vi "RT-Remote-v4.vi"() -> ()   [LabVIEW 2017]
uses:
  <vilib>/rvi/interface/nirviOpenFPGA/nirviOpenFPGA.xnode
  <vilib>/rvi/interface/nirviMethod/nirviMethod.xnode
  <vilib>/rvi/interface/nirviCloseFPGA/nirviCloseFPGA.xnode
  <vilib>/rvi/interface/nirviReadWriteControl/nirviReadWriteControl.xnode
  <vilib>/rvi/interface/Simulation/niFpgaSimulationCallBeginRW.vi
  <vilib>/rvi/errors/niLvFpgaAdjustHostInterfaceError.vi
  <vilib>/FPGAPlugInAG/Dynamic/niLvFpga_WriteFifo_Dynamic.vi
  <vilib>/rvi/errors/niLvFpgaMergeErrorWithErrorCode.vi
  <vilib>/FPGAPlugInAG/Dynamic/niLvFpga_Reset_Dynamic.vi
  <vilib>/nisyscfg/nisyscfg.lvlib
  NiFpgaLv.dll
  State Machine.vi
  <vilib>/FPGAPlugInAG/cRIO-9068/niLvFpga_Open_cRIO-9068.vi
  <vilib>/rvi/interface/common/dynamic/niFpgaDynamicAddResources.vi
  <vilib>/FPGAPlugInAG/Dynamic/niLvFpga_Close_Dynamic.vi
  <vilib>/rvi/interface/nirviMethod/StockFPGA_InlinedMethodWaitForSingleIRQ.vi
  <vilib>/FPGAPlugInAG/Dynamic/niLvFpga_WaitOnIrq_Dynamic.vi
  <vilib>/FPGAPlugInAG/Dynamic/niLvFpga_AcknowledgeIrq_Dynamic.vi
  <vilib>/FPGAPlugInAG/Dynamic/niLvFpga_ReadFifo_Dynamic.vi
  FPGA Bitfiles/NIcRIOFPGA_OMX-TFPGA_FPGAoptimizeperf_aoKWFa4HCLY.lvbitx
panel:
  out "error before tcp read":errorcluster
  out "Error after tcp read":errorcluster
  in  "Reset RT":bool
  out "cluster 406":T1
  out "output cluster 406":cluster{u16, u16}
  out "data out 200":string
  out "data out 100":string
  out "RT-host IP":string="10.6.19.12"
  out "Master Computer IP":string="10.6.19.11"
  out "UDP refresh rate":u16=100
  out "UDP receiving port":i32=6666
  out "UDP sending port":u16=6666
  out "Run Status reporter":bool=TRUE
  out "JSON Command":string
  out "Command \nConnection Port":u16=5000
  out "error out":errorcluster
  out "RT-host Action State":T2(ring)
  out "RT-host\nMain State":T3(ring)
  out "JSON string":string
  in  "Temperature Units (C) 2":u16(ring) items=["Celsius", "Fahrenheit", "Kelvin", "Rankine"]
  in  "ThermocoupleType 2":u16(ring)=2 items=["B", "E", "J", "K", "R", "S", "T", "N", "IC (C)", "IC (F)", "Therm."]
  out "Data sender Error out":errorcluster caption="error out"
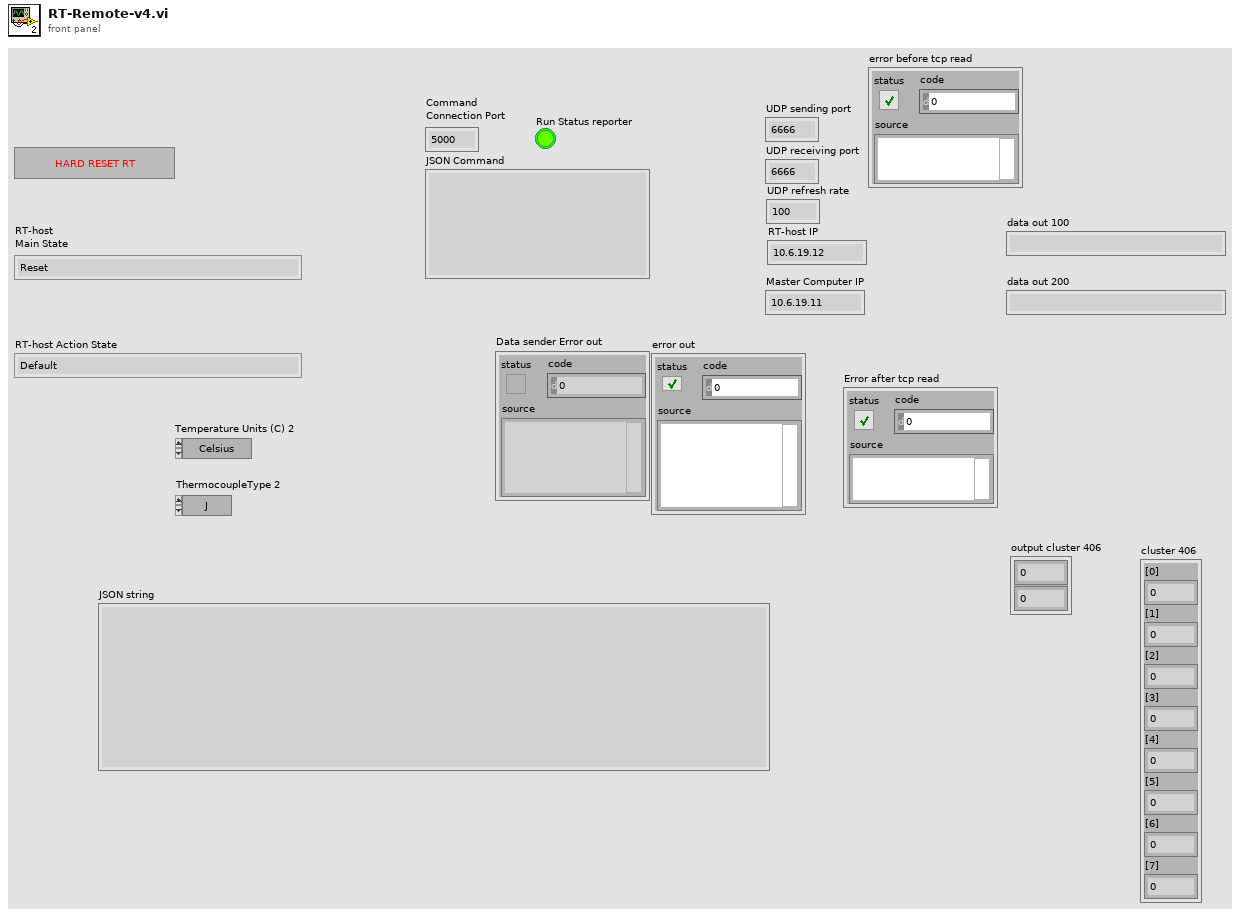
[diagram p1: front panel]
types:
  T1 = cluster{"[0]":u16, "[1]":u16, "[2]":u16, "[3]":u16, "[4]":u16, "[5]":u16, "[6]":u16, "[7]":u16}
  T2 = enum16{"Default", "Sending Digitals", "Sending Analogue", "Writing Digitals", "Writing Analogue", "Updating Repetitions", "Updating Indexes", "Init Profile", "Triggering Experiment", "Take Snap", "Flushing FIFOs", ""}
  T3 = enum16{"Reset", "Start", "Configuring", "Waiting Connection", "Idle", "Verifying FPGA state", "Sending Sync Command", "Sending Async Command", "Aborted", "Shutdown"}
  T4 = cluster{"Command":u16, "Message Length":u16, "Number of Messages":u32}
  T5 = enum16{"Reset", "Start", "Configuring", "Waiting Connection", "Idle", "Verifying FPGA state", "Sending Sync Command", "Sending Async Command", "Aborted", "Shutdown", "Send Error", ""}
  T6 = cluster{"FPGA Main State":u8, "FPGA Action State":u8, "Digitals":u16, "Analogue 0":i16, "Analogue 1":i16, "Analogue 2":i16, "Analogue 3":i16, "Temperature 0":sgl, "Temperature 1":sgl, "Temperature 2":sgl, "Temperature 3":sgl, "Error Description":string, "Error Status":bool, "Error code":i32, "RT-host Main State":u8, "RT-host Action State":u8, "Aborted":bool, "Interlock":bool, "Event":string}
  T7 = enum8{"Default", "Start", "Configuring", "Idle", "Aborted", "Running Action", "ShutDown"}
  T8 = enum8{"Default", "Executing Experiment", "Transfering Digitals", "Transfering Analogues", "Writing Indexes", "Writing Digitals", "Writing Analogue", "Taking Snap", "Flushing FIFOs", "Updating Repetitions"}
  T9 = cluster{"Mod6/CJC":fxp<+/-,24,-2>, "Mod6/TC0":fxp<+/-,24,-2>, "Mod6/TC1":fxp<+/-,24,-2>, "Mod6/TC2":fxp<+/-,24,-2>, "Mod6/TC3":fxp<+/-,24,-2>, "Mod6/Autozero":fxp<+/-,24,-2>}
  T10 = cluster{"Command":u8, "Message Length":u16, "Number of Messages":u32}
  T11 = enum16{"Standard", "Buffered", "CRLF", "Immediate"}
  T12 = cluster{"Command":u8, "Message Length":u16, "Number of Messages":u16}
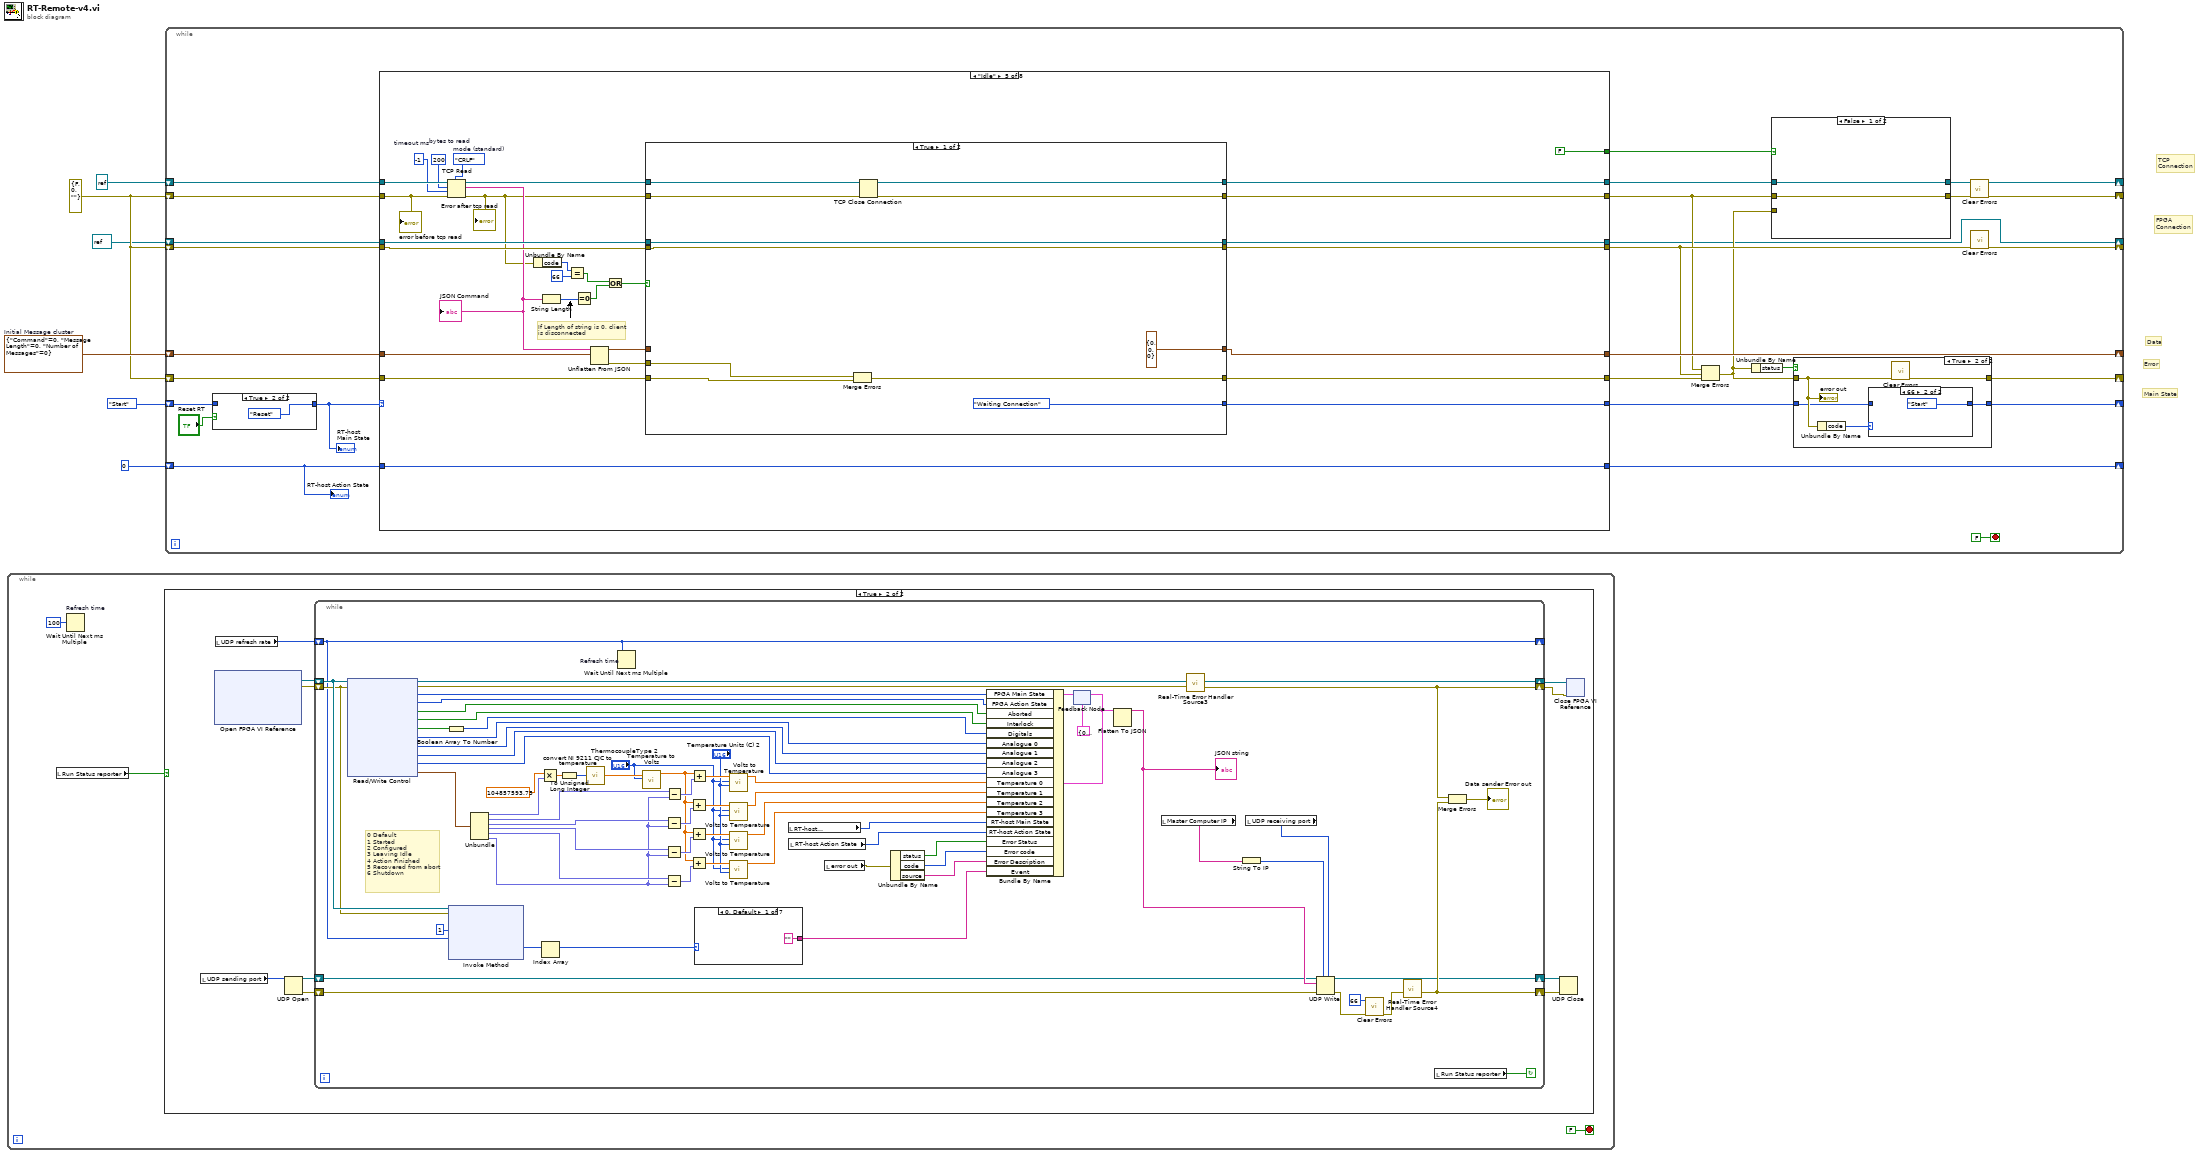
[diagram p0: block diagram]
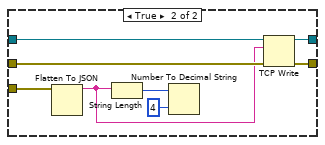
[diagram p3: hidden frame]
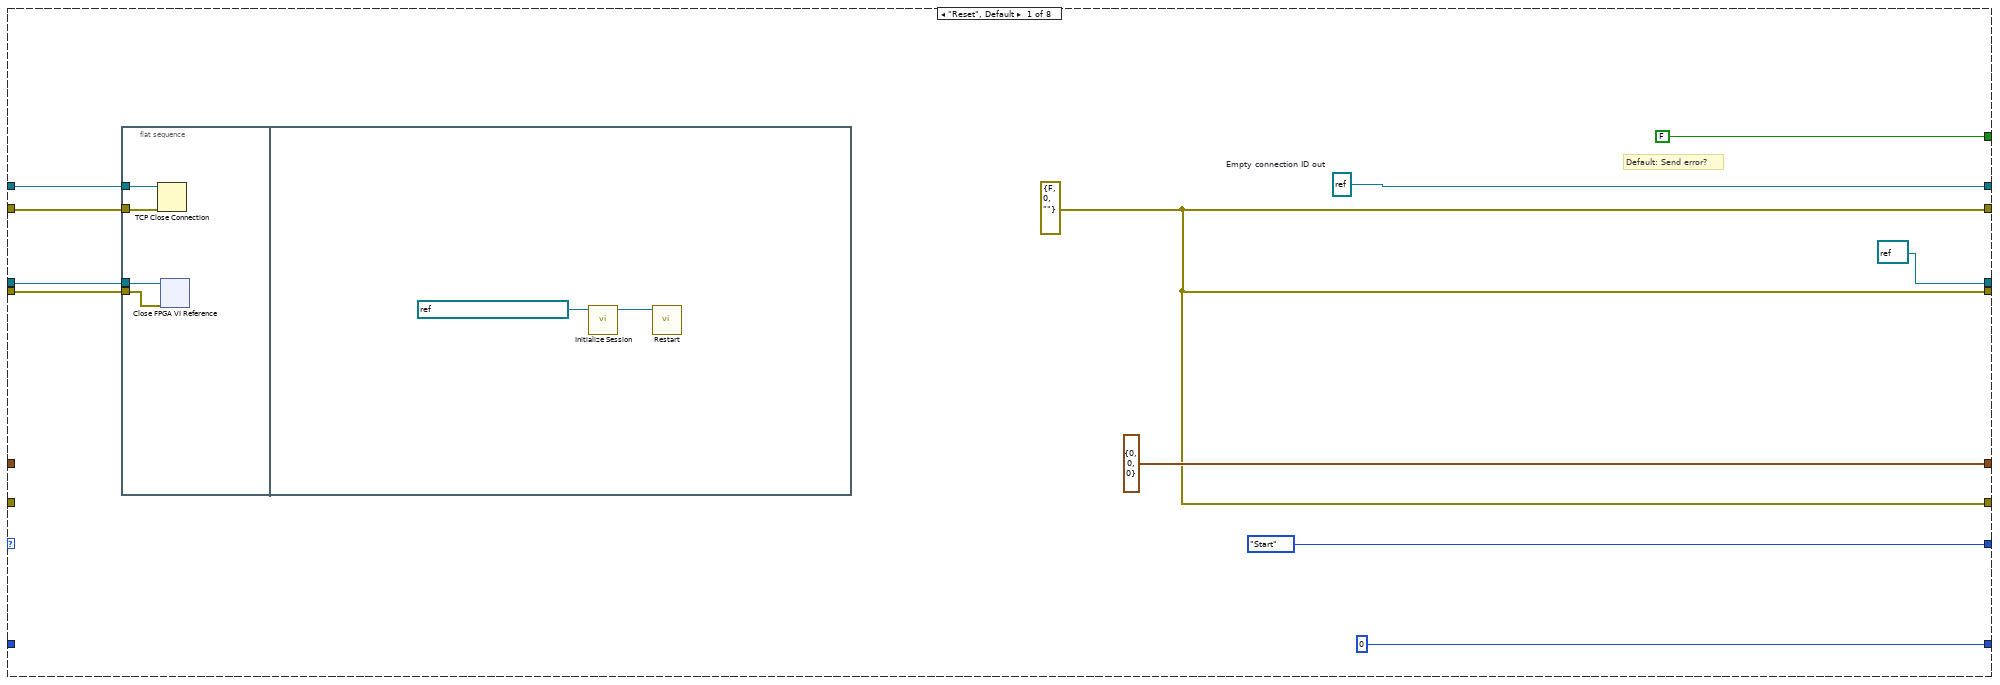
[diagram p6: hidden frame]
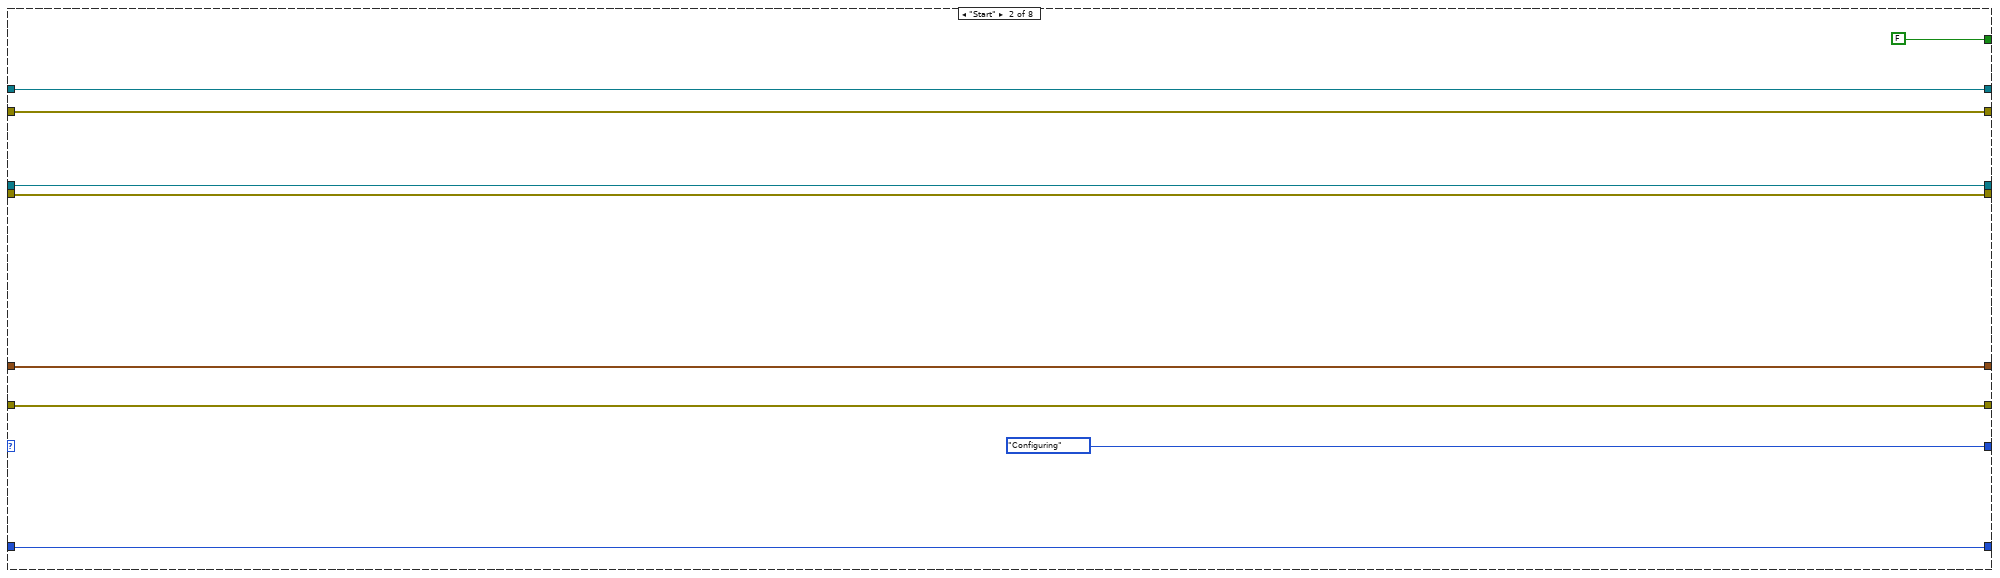
[diagram p7: hidden frame]
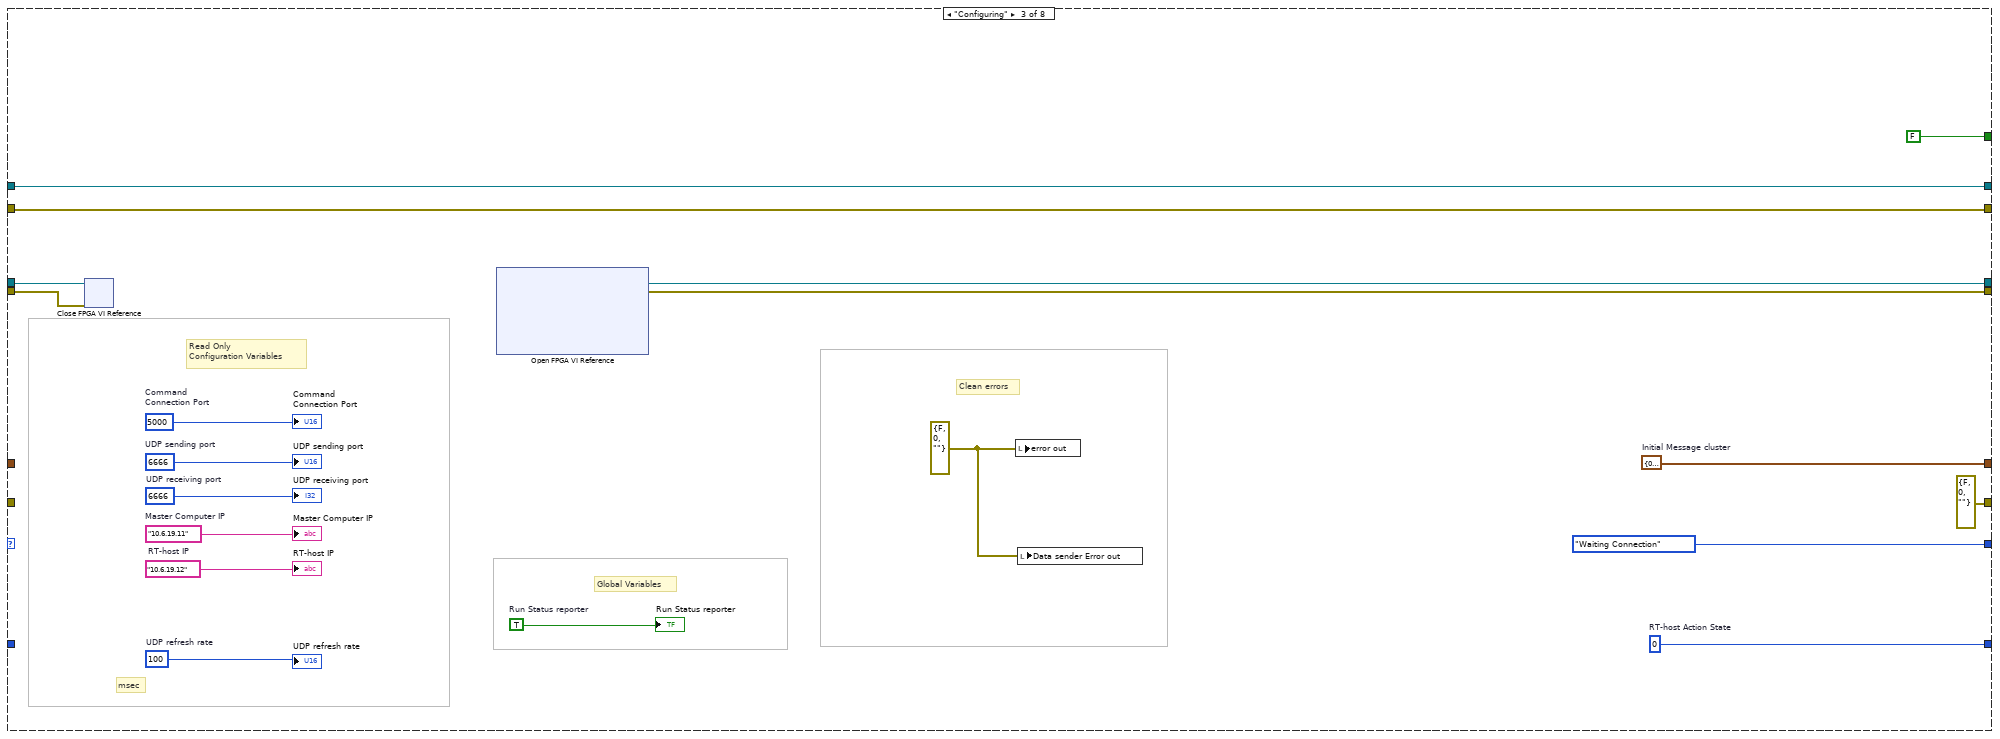
[diagram p8: hidden frame]
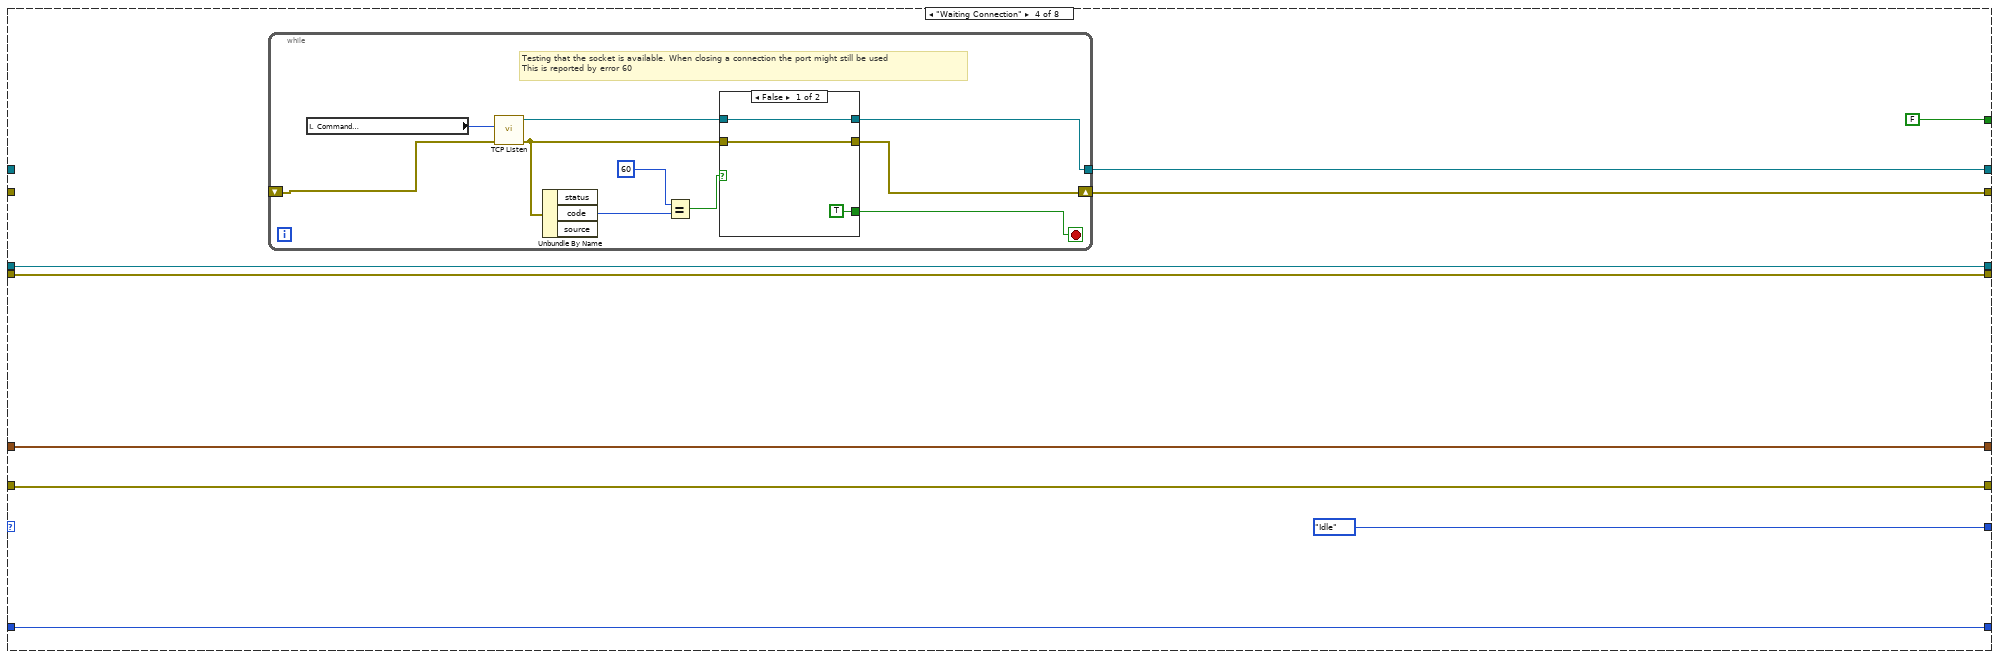
[diagram p9: hidden frame]
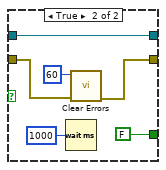
[diagram p10: hidden frame]
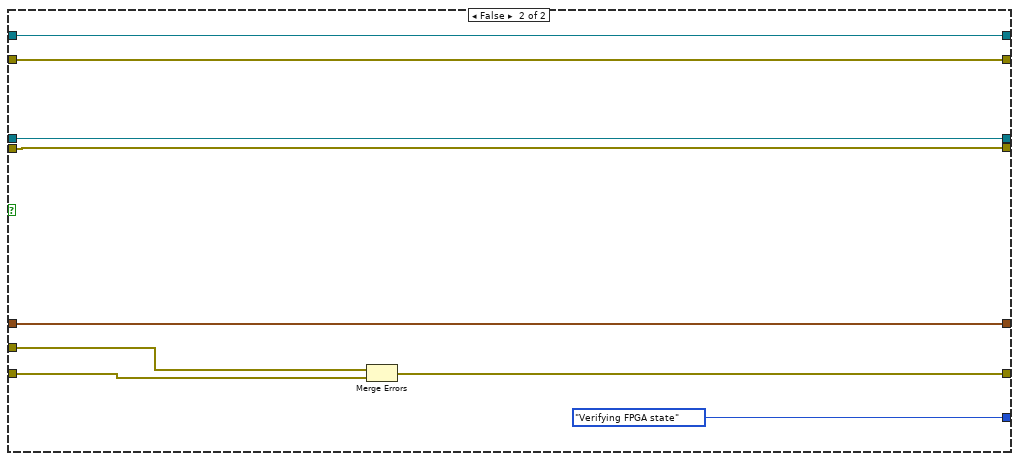
[diagram p11: hidden frame]
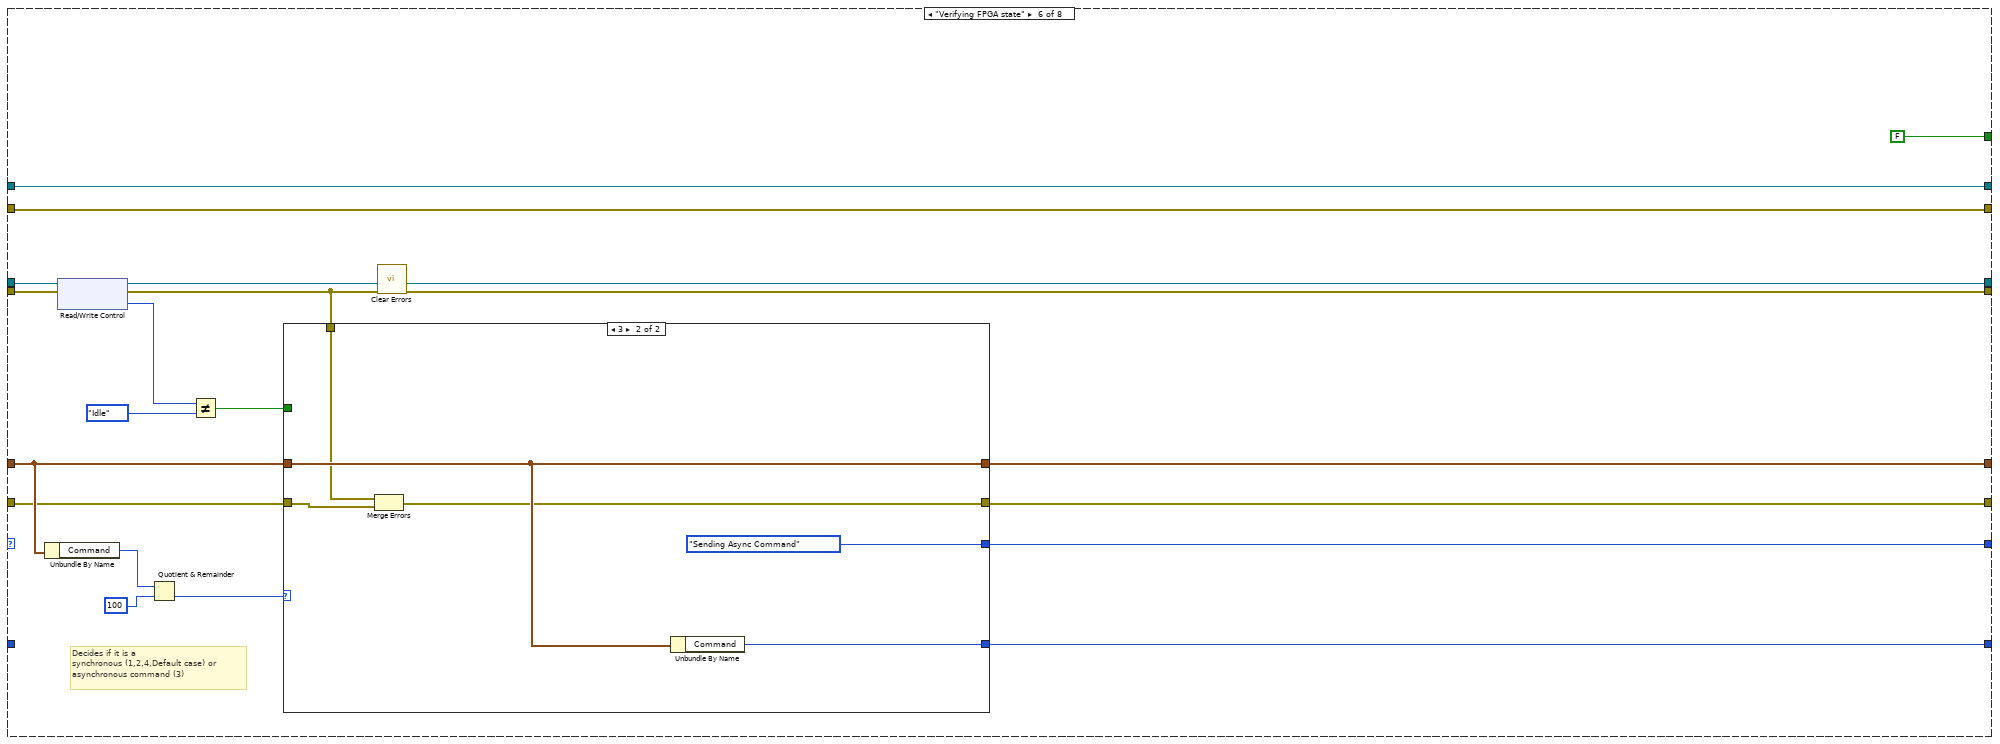
[diagram p12: hidden frame]
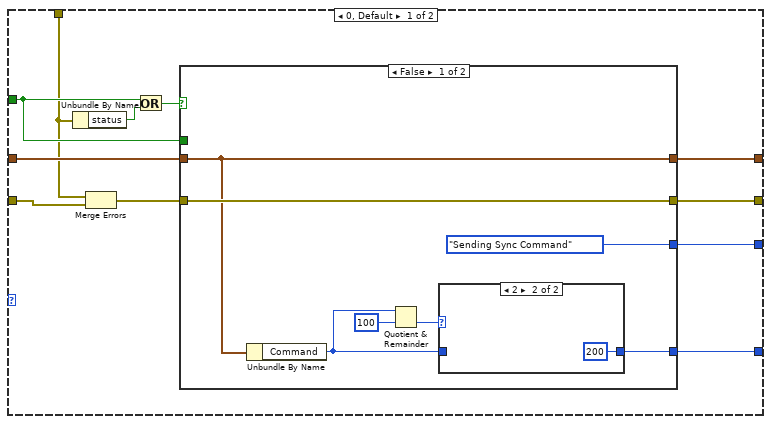
[diagram p13: hidden frame]
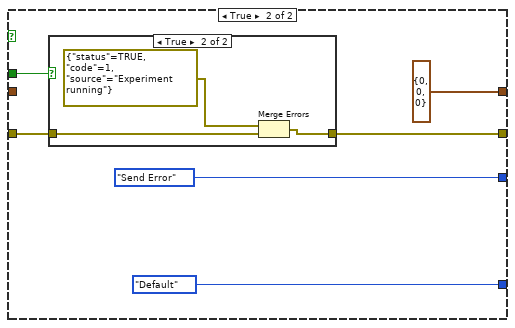
[diagram p15: hidden frame]
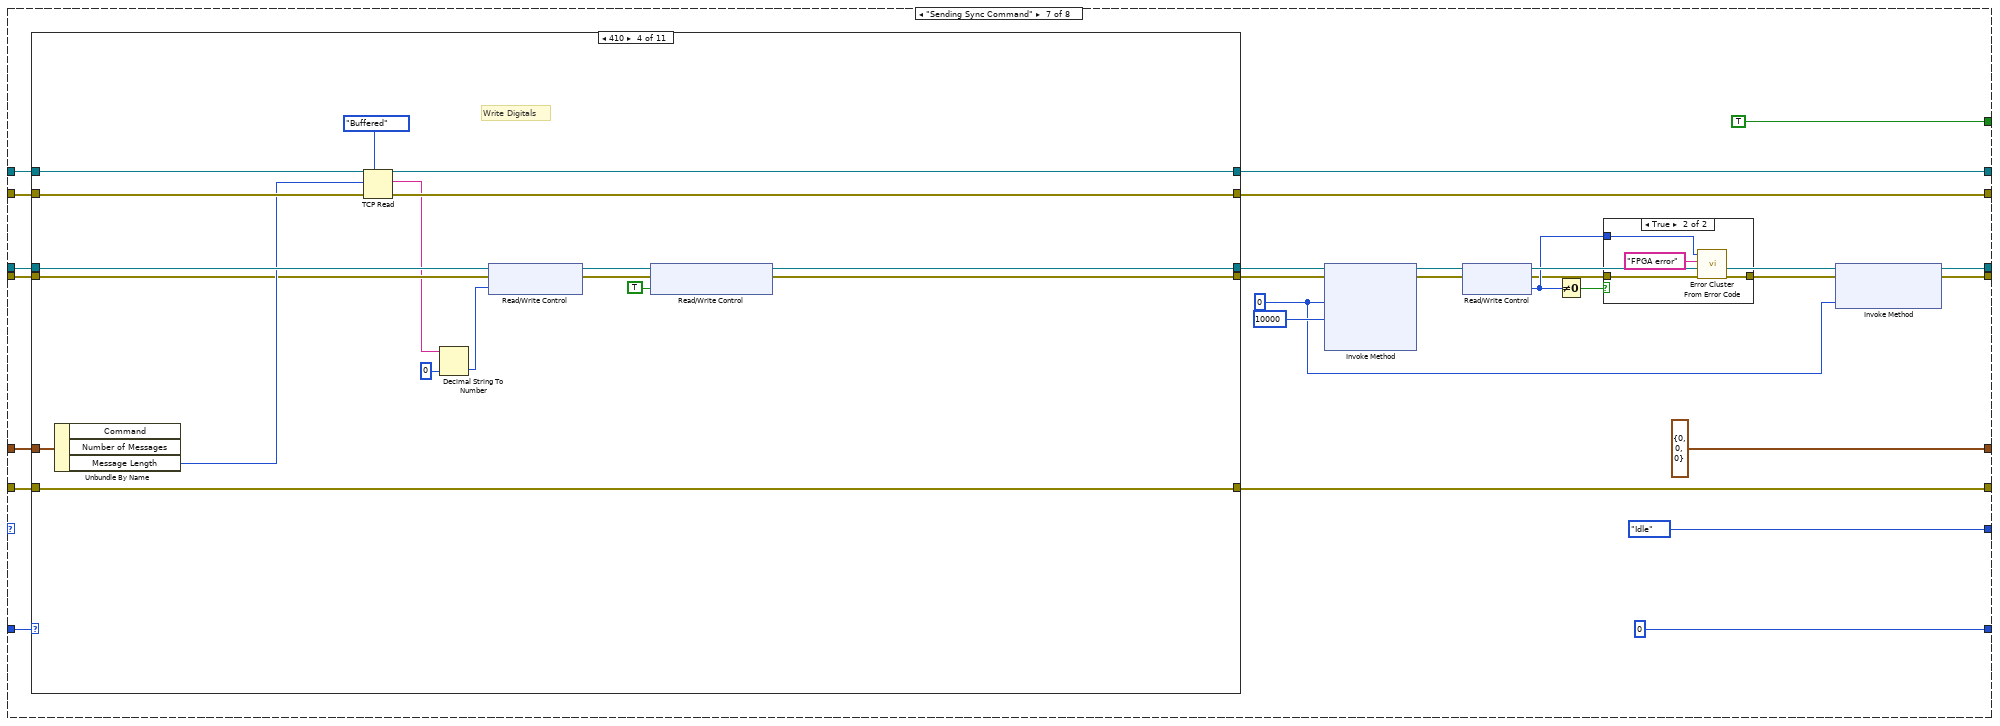
[diagram p17: hidden frame]
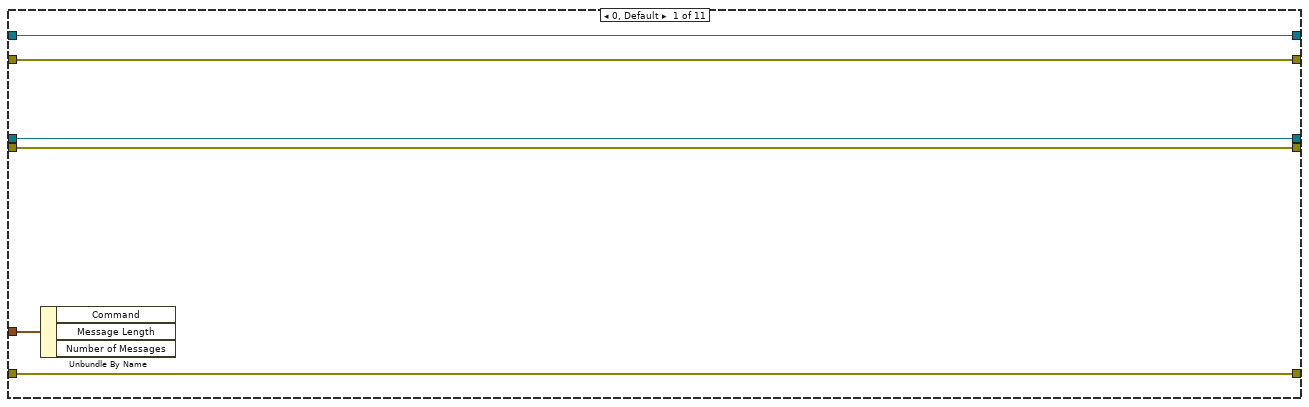
[diagram p19: hidden frame]
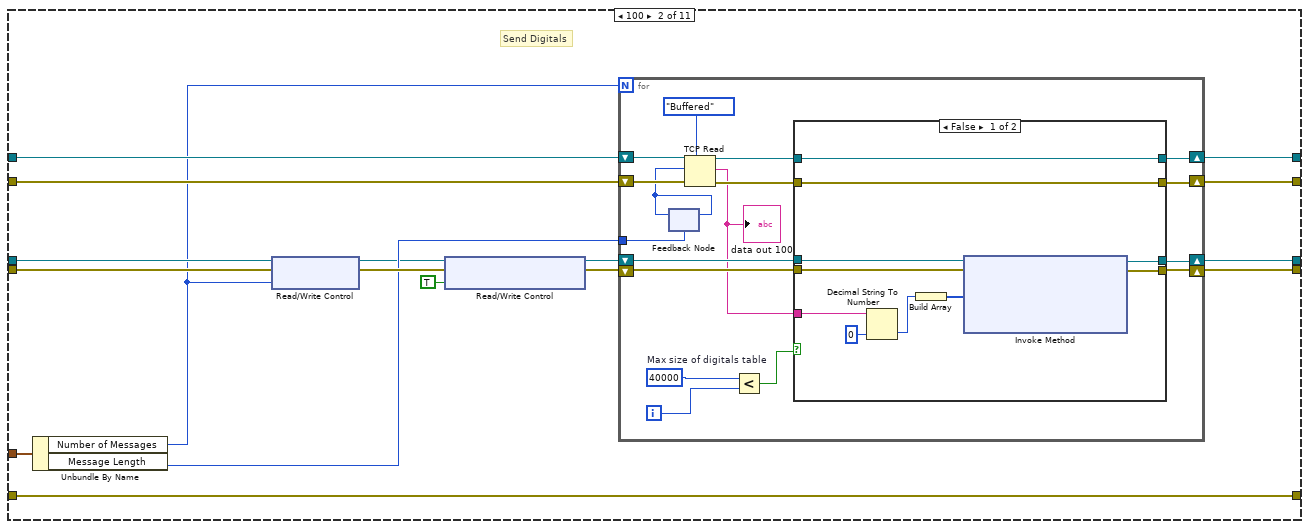
[diagram p20: hidden frame]
diagram:
  w2 = errorcluster {"status"=FALSE, "code"=0, "source"=""} ("error out")
  w5 = T4 {"Command"=0, "Message Length"=0, "Number of Messages"=0}  # Initial Message cluster
  # "Main State"
  # "Error"
  # "Data"
  # "FPGA\nConnection"
  # "TCP\nConnection"
  n1 = while {
    stop <- FALSE stop-if-true
    n2 = local read "Run Status reporter"() -> (w7:bool)
    n3 = Wait Until Next ms Multiple "Refresh time"(millisecond multiple=u32 100) -> ()  [unwired: 1 out]
    n4 = case shown="True" w7 {
      frame False {
      }
      frame True {
        n5 = local read "UDP sending port"() -> (w11:u16)
        n6 = xnode "Open FPGA VI Reference"() -> ("FPGA VI Reference Out"=w12:refnum<k20>, "error out"=w13:errorcluster)  [unwired: 2 in]
        n7 = local read "UDP refresh rate"() -> (w10:u16)
        n8 = UDP Open(11:w11) -> (port=w17:refnum<k16>, 0:w14:errorcluster)  [unwired: 4 in, 1 out]
        n9 = while {
          shift-right: [w84] -> w16
          shift-left: w17 -> [w22]
          shift-right: [w85] -> w18
          shift-left: w14 -> [w21]
          shift-right: [w56] -> w19
          shift-left: w12 -> [w30]
          shift-right: [w83] -> w15
          shift-left: w13 -> [w26]
          shift-right: [w24] -> _
          shift-left: w10 -> [w24]
          stop <- w32 continue-if-true
          # "0 Default\n1 Started\n2 Configured\n3 Leaving Idle \n4 Action Finished\n5 Recovered from abort\n6 Shutdown"
          n10 = xnode "Read/Write Control"("FPGA VI Reference In"=w30, "error in"=w26) -> ("FPGA VI Reference Out"=w56:refnum<k20>, "error out"=w55:errorcluster, "Main State"=w44:T7, "Action State"=w45:T8, "Aborted"=w34:bool, "Interlock"=w57:bool, "Digitals"=w80:bool[], "Analogue 0"=w47:i16, "Analogue 1"=w48:i16, "Analogue 2"=w49:i16, "Analogue 3"=w50:i16, "Temperatures array"=w58:T9)
          n11 = Boolean Array To Number(Boolean array=w80) -> (number=w46:u16)
          n12 = xnode "Invoke Method"("FPGA VI Reference In"=w30, "error in"=w26, "Number of Elements"=u32 1, "Timeout (ms)"=w24) -> ("Data"=w28:u8[])  [unwired: 3 out]
          n13 = Unbundle(w58) -> ("Mod6/CJC"=w76:fxp<+/-,24,-2>, "Mod6/TC0"=w73:fxp<+/-,24,-2>, "Mod6/TC1"=w66:fxp<+/-,24,-2>, "Mod6/TC2"=w65:fxp<+/-,24,-2>, "Mod6/TC3"=w64:fxp<+/-,24,-2>, "Mod6/Autozero"=w63:fxp<+/-,24,-2>)
          n14 = Multiply(x=104857593.75 ("y"), y=w76) -> (x*y=w77:dbl)
          n15 = Index Array(array=w28) -> (element=w27:u8)  [unwired: 1 in]
          n16 = To Unsigned Long Integer(number=w77) -> (unsigned 32bit integer=w78:u32)
          n17 = call "convert NI 9211 CJC to temperature.vi"("CJC Channel"=w78) -> ("CJC Temperature (C)"=w79:sgl)
          n18 = Wait Until Next ms Multiple "Refresh time"(millisecond multiple=w24) -> ()  [unwired: 1 out]
          n19 = call "Temperature to Volts.vi"("ThermocoupleType"="ThermocoupleType 2", "Temperature"=w79) -> ("Thermocouple Voltage"=w59:sgl)  [unwired: 1 in, 4 out]
          n20 = Subtract(x=w66, y=w63) -> (x-y=w62:fxp<+/-,25,-1>)
          n21 = Subtract(x=w65, y=w63) -> (x-y=w61:fxp<+/-,25,-1>)
          n22 = Subtract(x=w64, y=w63) -> (x-y=w60:fxp<+/-,25,-1>)
          n23 = Subtract(x=w73, y=w63) -> (x-y=w72:fxp<+/-,25,-1>)
          n24 = Add(x=w59, y=w62) -> (x+y=w71:sgl)
          n25 = Add(x=w59, y=w61) -> (x+y=w70:sgl)
          n26 = Add(x=w59, y=w60) -> (x+y=w69:sgl)
          n27 = Add(x=w59, y=w72) -> (x+y=w74:sgl)
          n28 = case shown="0, Default" w27 {
            tunnel: ["" "started" "configured" "leaving idle" "done" "recovered from abort" "shutdown"] -> w25
            frame 0, Default {
            }
            frame 1 {
            }
            frame 2 {
            }
            frame 3 {
            }
            frame 4 {
            }
            frame 5 {
            }
            frame 6 {
            }
          }
          n29 = call <vilib>:"Volts to Temperature.vi"("Temperature Units"="Temperature Units (C) 2", "ThermocoupleType"="ThermocoupleType 2", "Thermocouple Voltage"=w71) -> ("Temperature"=w52:sgl)  [unwired: 4 out]
          n30 = call <vilib>:"Volts to Temperature.vi"("Temperature Units"="Temperature Units (C) 2", "ThermocoupleType"="ThermocoupleType 2", "Thermocouple Voltage"=w70) -> ("Temperature"=w53:sgl)  [unwired: 4 out]
          n31 = call <vilib>:"Volts to Temperature.vi"("Temperature Units"="Temperature Units (C) 2", "ThermocoupleType"="ThermocoupleType 2", "Thermocouple Voltage"=w69) -> ("Temperature"=w54:sgl)  [unwired: 4 out]
          n32 = call <vilib>:"Volts to Temperature.vi"("Temperature Units"="Temperature Units (C) 2", "ThermocoupleType"="ThermocoupleType 2", "Thermocouple Voltage"=w74) -> ("Temperature"=w51:sgl)  [unwired: 4 out]
          n33 = local read "RT-host\nMain State"() -> (w40:T3)
          n34 = local read "RT-host Action State"() -> (w39:T2)
          n35 = local read "error out"() -> (w38:errorcluster)
          n36 = Unbundle By Name(w38) -> ("status"=w37:bool, "code"=w36:i32, "source"=w35:string)
          n37 = feedback #1(T6 {"FPGA Main State"=0, "FPGA Action State"=0, "Digitals"=0, "Analogue 0"=0, "Analogue 1"=0, "Analogue 2"=0, "Analogue 3"=0, "Temperature 0"=0.0, "Temperature 1"=0.0, "Temperature 2"=0.0, "Temperature 3"=0.0, "Error Description"="", "Error Status"=FALSE, "Error code"=0, "RT-host Main State"=0, "RT-host Action State"=0, "Aborted"=FALSE, "Interlock"=FALSE, "Event"=""}) -> (w42:T6)
          n38 = Bundle By Name(cluster=w42, "FPGA Main State"=w44, "FPGA Action State"=w45, "Aborted"=w34, "Interlock"=w57, "Digitals"=w46, "Analogue 0"=w47, "Analogue 1"=w48, "Analogue 2"=w49, "Analogue 3"=w50, "Temperature 0"=w51, "Temperature 1"=w52, "Temperature 2"=w53, "Temperature 3"=w54, "RT-host Main State"=w40, "RT-host Action State"=w39, "Error Status"=w37, "Error code"=w36, "Error Description"=w35, "Event"=w25) -> (w41:T6)
          n39 = feedback-in #1(w41) -> ()
          n40 = Flatten To JSON(anything=w41) -> (JSON string=w31:string)  [unwired: 2 in, 1 out]
          "JSON string" <- w31
          n41 = local read "Master Computer IP"() -> (w33:string)
          n42 = call "Real-Time Error Handler Source3"("Error to Check"=w55) -> ("error out"=w83:errorcluster)  [unwired: 11 in, 3 out]
          n43 = String To IP(1:w33) -> (0:w23:u32)
          n44 = local read "UDP receiving port"() -> (w20:i32)
          n45 = UDP Write(address=w23, port or service name=w20, connection ID=w22, data in=w31, 8:w21) -> (error out=w87:errorcluster, 3:w84:refnum<k16>)  [unwired: 1 in]
          n46 = call <vilib>:"Clear Errors.vi"("error in (no error)"=w87, "specific error code to clear (0: all)"=66) -> ("error out"=w82:errorcluster)  [unwired: 4 in, 1 out]
          n47 = call "Real-Time Error Handler Source4"("Error to Check"=w82) -> ("error out"=w85:errorcluster)  [unwired: 11 in, 3 out]
          n48 = local read "Run Status reporter"() -> (w32:bool)
          n49 = Merge Errors(w83, w85) -> (→"Data sender Error out":errorcluster)
        }
        n50 = UDP Close(connection ID=w16, 8:w18) -> ()  [unwired: 2 out]
        n51 = xnode "Close FPGA VI Reference"("FPGA VI Reference In"=w19, "error in"=w15) -> ()  [unwired: 1 out]
      }
    }
  }
  n52 = while {
    shift-right: [w100] -> _
    shift-left: T5."Start" ("RT-host Main State") -> [w97]
    shift-right: [w105] -> _
    shift-left: refnum<k5> refnum ("connection ID out") -> [w122]
    shift-right: [w121] -> _
    shift-left: w5 -> [w120]
    shift-right: [w118] -> _
    shift-left: u16 0 ("RT-host Action State") -> [w115]
    shift-right: [w111] -> _
    shift-left: w2 -> [w117]
    shift-right: [w110] -> _
    shift-left: w2 -> [w116]
    shift-right: [w113] -> _
    shift-left: w2 -> [w114]
    shift-right: [w98] -> _
    shift-left: refnum<k20> refnum ("FPGA VI Reference Out") -> [w99]
    stop <- FALSE stop-if-true
    n53 = case shown="True" "Reset RT" {
      tunnel: [w123 T5."Reset" ("RT-host Main State")] -> w96
      tunnel: w97 -> [w123 _]
      frame False {
      }
      frame True {
      }
    }
    "RT-host\nMain State" <- w96
    n54 = case shown="\"Idle\"" w96 {
      tunnel: [refnum<k20> refnum ("FPGA VI Reference Out") w161 w175 w189 w230 w265 w325 w655] -> w98
      tunnel: [w152 w167 w185 w197 w233 w284 w333 w670] -> w106
      tunnel: [w150 w163 errorcluster {"status"=FALSE, "code"=0, "source"=""} ("error out") w192 w240 w277 w332 w660] -> w112
      tunnel: w122 -> [w149 w167 w185 _ w244 w284 w346 w669]
      tunnel: [T5."Start" ("RT-host Main State") T3."Configuring" ("RT-host Main State") T3."Waiting Connection" ("RT-host Main State") T3."Idle" ("RT-host Main State") w245 w278 T5."Idle" ("RT-host Main State") w662] -> w101
      tunnel: [T10 {"Command"=0, "Message Length"=0, "Number of Messages"=0} ("Initial Message cluster") w164 w187 w195 w226 w275 T10 {"Command"=0, "Message Length"=0, "Number of Messages"=0} ("Initial Message cluster") T10 {"Command"=0, "Message Length"=0, "Number of Messages"=0} ("Initial Message cluster")] -> w121
      tunnel: w120 -> [_ w164 _ w195 w236 w272 w342 w665]
      tunnel: w115 -> [_ w168 _ w194 w239 _ w347 w671]
      tunnel: [u16 0 ("RT-host Action State") w168 w186 w194 w239 w276 u16 0 ("RT-host Action State") u16 0 ("RT-host Action State")] -> w118
      tunnel: [w150 w165 w174 w193 w229 w268 w323 w654] -> w109
      tunnel: w117 -> [w146 w165 w173 w193 w228 w281 w343 w666]
      tunnel: [w150 w166 w184 w191 w232 w280 w334 w658] -> w108
      tunnel: w116 -> [w148 w166 w184 _ w238 w280 w345 w668]
      tunnel: w114 -> [_ w163 _ w192 w237 w269 w341 w664]
      tunnel: [FALSE FALSE FALSE FALSE FALSE FALSE TRUE TRUE] -> w103
      tunnel: w99 -> [w145 w161 w170 w189 w231 w266 w321 w651]
      frame "Reset", Default {
        w152 = refnum<k5> refnum  # Empty connection ID out
        w150 = errorcluster {"status"=FALSE, "code"=0, "source"=""} ("error out")
        # "Default: Send error?"
        n55 = flat-sequence {
          tunnel: w149 -> [w158]
          tunnel: w148 -> [w157]
          tunnel: w146 -> [w156]
          tunnel: w145 -> [w155]
          frame #0 {
            n56 = TCP Close Connection(connection ID=w158, error in (no error)=w157) -> ()  [unwired: 1 in, 2 out]
            n57 = xnode "Close FPGA VI Reference"("FPGA VI Reference In"=w155, "error in"=w156) -> ()  [unwired: 1 out]
          }
          frame #1 {
            n58 = call <vilib>:"Initialize Session.vi"("Target (localhost)"=refnum<k21> "NI-cRIO-9068 (10.6.19.12)") -> ("Session out"=w159:refnum<k21>)  [unwired: 9 in, 1 out]
            n59 = call <vilib>:"Restart.vi"("Session in"=w159) -> ()  [unwired: 8 in, 3 out]
          }
        }
      }
      frame "Start" {
      }
      frame "Configuring" {
        w176 = errorcluster {"status"=FALSE, "code"=0, "source"=""} ("error out")
        w178 = TRUE  # Run Status reporter
        w183 = 6666  # UDP receiving port
        w182 = u16 100  # UDP refresh rate
        w181 = "10.6.19.12"  # RT-host IP
        w180 = "10.6.19.11"  # Master Computer IP
        w179 = u16 6666  # UDP sending port
        w177 = u16 5000  # Command  Connection Port
        w186 = 0  # RT-host Action State
        w187 = T12 {"Command"=0, "Message Length"=0, "Number of Messages"=0}  # Initial Message cluster
        # "Clean errors"
        # "Global Variables"
        # "msec"
        # "Read Only\nConfiguration Variables"
        n60 = xnode "Close FPGA VI Reference"("FPGA VI Reference In"=w170, "error in"=w173) -> ()  [unwired: 1 out]
        n61 = xnode "Open FPGA VI Reference"() -> ("FPGA VI Reference Out"=w175:refnum<k20>, "error out"=w174:errorcluster)  [unwired: 2 in]
        n62 = local write "error out"(w176) -> ()
        n63 = local write "Data sender Error out"(w176) -> ()
        "Command \nConnection Port" <- w177
        "Run Status reporter" <- w178
        "UDP sending port" <- w179
        "UDP receiving port" <- w183
        "UDP refresh rate" <- w182
        "Master Computer IP" <- w180
        "RT-host IP" <- w181
      }
      frame "Waiting Connection" {
        n64 = while {
          tunnel: [w201] -> w197
          shift-right: [w204] -> w191
          shift-left: _ -> [w198]
          stop <- w199 stop-if-true
          # "Testing that the socket is available. When closing a connection the port might still be used\nThis is reported by error 60"
          n65 = local read "Command \nConnection Port"() -> (w207:u16)
          n66 = call <vilib>:"TCP Listen.vi"("error in (no error)"=w198, "port"=w207) -> ("error out"=w203:errorcluster, "connection ID"=w200:refnum<k5>)  [unwired: 5 in, 3 out]
          n67 = Unbundle By Name(w203) -> ("code"=w206:i32)  [unwired: 2 out]
          n68 = Equal?(x=60, y=w206) -> (x = y?=w202:bool)
          n69 = case shown="False" w202 {
            tunnel: [w209 w214] -> w204
            tunnel: w203 -> [w209 w215]
            tunnel: [w210 w212] -> w201
            tunnel: w200 -> [w210 w212]
            tunnel: [TRUE FALSE] -> w199
            frame False {
            }
            frame True {
              n70 = Wait (ms)(milliseconds to wait=u32 1000) -> ()  [unwired: 1 out]
              n71 = call <vilib>:"Clear Errors.vi"("error in (no error)"=w215, "specific error code to clear (0: all)"=60) -> ("error out"=w214:errorcluster)  [unwired: 4 in, 1 out]
            }
          }
        }
      }
      frame "Idle" {
        w223 = 200  # bytes to read
        w242 = -1  # timeout ms
        w243 = T11."CRLF"  # mode (standard)
        # "If Length of string is 0, client\nis disconnected"
        n72 = TCP Read(connection ID=w244, bytes to read=w223, error in (no error)=w238, 7:w243, 9:w242) -> (connection ID out=w234:refnum<k5>, data out=w225:string, error out=w221:errorcluster)
        "JSON Command" <- w225
        "Error after tcp read" <- w221
        n73 = Unbundle By Name(w221) -> ("code"=w222:i32)
        n74 = String Length(string=w225) -> (length=w224:i32)
        n75 = Equal?(x=w222, y=66) -> (x = y?=w219:bool)
        n76 = Equal To 0?(x=w224) -> (x = 0?=w218:bool)
        n77 = Unflatten From JSON(JSON string=w225, type and defaults=w236) -> (value=w227:T4, error out=w241:errorcluster)  [unwired: 5 in]
        n78 = Or(x=w219, y=w218) -> (x .or. y?=w217:bool)
        n79 = case shown="True" w217 {
          tunnel: [T3."Waiting Connection" ("RT-host Main State") T3."Verifying FPGA state" ("RT-host Main State")] -> w245
          tunnel: w241 -> [w254 w263]
          tunnel: [w253 w262] -> w240
          tunnel: w237 -> [w252 w261]
          tunnel: w234 -> [w251 w260]
          tunnel: [w246 w260] -> w233
          tunnel: [w250 w259] -> w232
          tunnel: w221 -> [w250 w259]
          tunnel: w231 -> [w249 w258]
          tunnel: [w249 w258] -> w230
          tunnel: [w248 w257] -> w229
          tunnel: w228 -> [w248 w257]
          tunnel: w227 -> [_ w256]
          tunnel: [T4 {"Command"=0, "Message Length"=0, "Number of Messages"=0} ("Initial Message cluster") w256] -> w226
          frame True {
            n80 = Merge Errors(w254, w252) -> (w253:errorcluster)
            n81 = TCP Close Connection(connection ID=w251) -> (connection ID out=w246:refnum<k5>)  [unwired: 2 in, 1 out]
          }
          frame False {
            n82 = Merge Errors(w263, w261) -> (w262:errorcluster)
          }
        }
        "error before tcp read" <- w238
      }
      frame "Verifying FPGA state" {
        # "Decides if it is a \nsynchronous (1,2,4,Default case) or\nasynchronous command (3)"
        n83 = Unbundle By Name(w272) -> ("Command"=w271:u16)
        n84 = xnode "Read/Write Control"("FPGA VI Reference In"=w266, "error in"=w281) -> ("FPGA VI Reference Out"=w265:refnum<k20>, "error out"=w279:errorcluster, "Main State"=w283:T7)
        n85 = Quotient & Remainder(x=w271, y=100) -> (floor(x/y)=w273:i32)  [unwired: 1 out]
        n86 = Not Equal?(x=w283, y=T7."Idle") -> (x != y?=w270:bool)
        n87 = case shown="3" w273 {
          tunnel: w279 -> [w287 w317]
          tunnel: [w295 T3."Sending Async Command" ("RT-host Main State")] -> w278
          tunnel: [w294 w316] -> w277
          tunnel: [w293 w319] -> w276
          tunnel: [w292 w318] -> w275
          tunnel: w272 -> [w291 w318]
          tunnel: w270 -> [w288 _]
          tunnel: w269 -> [w285 w315]
          frame 0, Default {
            n88 = Unbundle By Name(w287) -> ("status"=w289:bool)
            n89 = Merge Errors(w287, w285) -> (w286:errorcluster)
            n90 = Or(x=w288, y=w289) -> (x .or. y?=w290:bool)
            n91 = case shown="False" w290 {
              tunnel: [T3."Sending Sync Command" ("RT-host Main State") T5."Send Error" ("RT-host Main State")] -> w295
              tunnel: w286 -> [w301 w307]
              tunnel: [w301 w306] -> w294
              tunnel: [w299 T2."Default" ("RT-host Action State")] -> w293
              tunnel: [w300 T10 {"Command"=0, "Message Length"=0, "Number of Messages"=0} ("Initial Message cluster")] -> w292
              tunnel: w291 -> [w300 _]
              tunnel: w288 -> [_ w305]
              frame False {
                n92 = Unbundle By Name(w300) -> ("Command"=w297:u16)
                n93 = Quotient & Remainder(x=w297, y=u16 100) -> (floor(x/y)=w298:u16)  [unwired: 1 out]
                n94 = case shown="2" w298 {
                  tunnel: [w303 u16 200 ("Command")] -> w299
                  tunnel: w297 -> [w303 _]
                  frame 0, Default {
                  }
                  frame 2 {
                  }
                }
              }
              frame True {
                n95 = case shown="True" w305 {
                  tunnel: w307 -> [w311 w314]
                  tunnel: [w311 w313] -> w306
                  frame False {
                  }
                  frame True {
                    n96 = Merge Errors(errorcluster {"status"=TRUE, "code"=1, "source"="Experiment running"} ("error out"), w314) -> (w313:errorcluster)
                  }
                }
              }
            }
          }
          frame 3 {
            n97 = Merge Errors(w317, w315) -> (w316:errorcluster)
            n98 = Unbundle By Name(w318) -> ("Command"=w319:u16)
          }
        }
        n99 = call <vilib>:"Clear Errors.vi"("error in (no error)"=w279) -> ("error out"=w268:errorcluster)  [unwired: 5 in, 1 out]
      }
      frame "Sending Sync Command" {
        w324 = 0 ("IRQ Number(s)")
        n100 = case shown="410" w347 {
          tunnel: [w358 w372 w418 w452 w471 w508 w531 w587 w612 w624 w648] -> w333
          tunnel: w346 -> [w358 w370 w426 w459 w473 w514 w533 w603 w612 w622 w648]
          tunnel: [w357 w371 w417 w453 w470 w500 w530 w585 w611 w623 w647] -> w334
          tunnel: w345 -> [w357 w369 w425 w458 w472 w513 w532 w602 w611 w621 w647]
          tunnel: [w356 w368 w415 w456 w476 w511 w527 w600 w609 w628 w645] -> w344
          tunnel: w321 -> [w356 w367 w427 w457 w469 w512 w525 w601 w610 w616 w646]
          tunnel: [w355 w362 w414 w455 w475 w510 w526 w599 w608 w627 w644] -> w327
          tunnel: w343 -> [w355 w365 w413 w448 w468 w505 w524 w594 w606 w625 w642]
          tunnel: w342 -> [w353 w373 w428 w460 w477 w515 w559 w604 w613 w629 w649]
          tunnel: [w354 w374 w429 w461 w478 w516 w560 w605 w614 w630 w650] -> w332
          tunnel: w341 -> [w354 w374 w429 w461 w478 w516 w560 w605 w614 w630 w650]
          frame 0, Default {
            n101 = Unbundle By Name(w353) -> ()  [unwired: 3 out]
          }
          frame 100 {
            # "Send Digitals"
            n102 = Unbundle By Name(w373) -> ("Number of Messages"=w359:u32, "Message Length"=w361:u16)
            n103 = xnode "Read/Write Control"("FPGA VI Reference In"=w367, "Nr of Digitals"=w359) -> ("FPGA VI Reference Out"=w360:refnum<k20>)  [unwired: 1 in, 1 out]
            n104 = xnode "Read/Write Control"("FPGA VI Reference In"=w360, "error in"=w365, "Trigger digitals transfer"=TRUE) -> ("FPGA VI Reference Out"=w366:refnum<k20>, "error out"=w364:errorcluster)
            n105 = for {
              N: w359 -> [_]
              shift-right: [w388] -> w372
              shift-left: w370 -> [w384]
              shift-right: [w387] -> w371
              shift-left: w369 -> [w383]
              shift-right: [w381] -> w362
              shift-left: w364 -> [w385]
              shift-right: [w389] -> w368
              shift-left: w366 -> [w386]
              tunnel: w361 -> [w376]
              i -> [w379]
              w380 = u16 40000  # Max size of digitals table
              n106 = feedback #2(w376) -> (w375:u16)
              n107 = feedback-in #2(w375) -> ()
              n108 = TCP Read(connection ID=w384, bytes to read=w375, error in (no error)=w383, 7:T11."Buffered" ("mode (standard)")) -> (connection ID out=w390:refnum<k5>, data out=w378:string, error out=w391:errorcluster)  [unwired: 1 in]
              "data out 100" <- w378
              n109 = Less?(x=w380, y=w379) -> (x < y?=w377:bool)
              n110 = case shown="False" w377 {
                tunnel: [w401 w407] -> w388
                tunnel: w390 -> [w401 w407]
                tunnel: [w400 w406] -> w387
                tunnel: w391 -> [w400 w406]
                tunnel: w386 -> [w399 w404]
                tunnel: w385 -> [w398 w405]
                tunnel: [w397 w404] -> w389
                tunnel: [w396 w403] -> w381
                tunnel: w378 -> [w395 _]
                frame False {
                  n111 = Decimal String To Number(string=w395, default (0L)=u64 0 ("default (0 I32)")) -> (number=w393:u64)  [unwired: 1 in, 1 out]
                  n112 = Build Array(w393) -> (w394:u64[])
                  n113 = xnode "Invoke Method"("FPGA VI Reference In"=w399, "error in"=w398, "Data"=w394) -> ("FPGA VI Reference Out"=w397:refnum<k20>, "error out"=w396:errorcluster)  [unwired: 1 in, 1 out]
                }
                frame True {
                  n114 = Merge Errors(w405, errorcluster {"status"=TRUE, "code"=0, "source"="Digitals table is full"} ("error in")) -> (w403:errorcluster)
                }
              }
            }
          }
          frame 200 {
            # "Send Analogues"
            n115 = Unbundle By Name(w428) -> ("Command"=w421:u16, "Number of Messages"=w408:u32, "Message Length"=w424:u16)
            n116 = Quotient & Remainder(x=w421, y=u8 100) -> (x-y*floor(x/y)=w419:u16)  [unwired: 1 out]
            n117 = xnode "Read/Write Control"("FPGA VI Reference In"=w427, "error in"=w413, "Memory to Write"=w419) -> ("FPGA VI Reference Out"=w410:refnum<k20>, "error out"=w412:errorcluster)
            n118 = xnode "Read/Write Control"("FPGA VI Reference In"=w410, "error in"=w412, "Nr of Analogues"=w408) -> ("FPGA VI Reference Out"=w409:refnum<k20>, "error out"=w411:errorcluster)
            n119 = xnode "Read/Write Control"("FPGA VI Reference In"=w409, "error in"=w411, "Trigger analogues transfer"=TRUE) -> ("FPGA VI Reference Out"=w423:refnum<k20>, "error out"=w422:errorcluster)
            n120 = for {
              N: w408 -> [_]
              shift-right: [w443] -> w417
              shift-left: w425 -> [w438]
              shift-right: [w442] -> w418
              shift-left: w426 -> [w439]
              shift-right: [w430] -> _
              shift-left: w424 -> [w430]
              shift-right: [w441] -> w415
              shift-left: w423 -> [w435]
              shift-right: [w436] -> w414
              shift-left: w422 -> [w440]
              n121 = TCP Read(connection ID=w439, bytes to read=w430, error in (no error)=w438, 7:T11."Buffered" ("mode (standard)")) -> (connection ID out=w442:refnum<k5>, data out=w434:string, error out=w443:errorcluster)  [unwired: 1 in]
              "data out 200" <- w434
              n122 = Decimal String To Number(string=w434, default (0L)=u64 0 ("default (0 I32)")) -> (number=w431:u64)  [unwired: 1 in, 1 out]
              n123 = Build Array(w431) -> (w432:u64[])
              n124 = xnode "Invoke Method"("FPGA VI Reference In"=w435, "error in"=w440, "Data"=w432) -> ("FPGA VI Reference Out"=w441:refnum<k20>, "error out"=w436:errorcluster)  [unwired: 1 in, 1 out]
            }
          }
          frame 410 {
            # "Write Digitals"
            n125 = Unbundle By Name(w460) -> ("Message Length"=w450:u16)  [unwired: 2 out]
            n126 = TCP Read(connection ID=w459, bytes to read=w450, error in (no error)=w458, 7:T11."Buffered" ("mode (standard)")) -> (connection ID out=w452:refnum<k5>, data out=w444:string, error out=w453:errorcluster)  [unwired: 1 in]
            n127 = Decimal String To Number(string=w444, default (0L)=u32 0 ("default (0 I32)")) -> (number=w445:u32)  [unwired: 1 in, 1 out]
            n128 = xnode "Read/Write Control"("FPGA VI Reference In"=w457, "error in"=w448, "digitals to write"=w445) -> ("FPGA VI Reference Out"=w449:refnum<k20>, "error out"=w447:errorcluster)
            n129 = xnode "Read/Write Control"("FPGA VI Reference In"=w449, "error in"=w447, "Trigger Write Digitals"=TRUE ("Digitals transfer done")) -> ("FPGA VI Reference Out"=w456:refnum<k20>, "error out"=w455:errorcluster)
          }
          frame 411 {
            # "Write Analogue"
            n130 = Unbundle By Name(w477) -> ("Number of Messages"=w465:u32, "Message Length"=w467:u16)  [unwired: 1 out]
            n131 = Divide(x=w465, y=u16 2) -> (x/y=w466:dbl)
            n132 = for {
              N: w466 -> [_]
              shift-right: [w498] -> w463
              shift-left: w469 -> [w495]
              shift-right: [w497] -> w462
              shift-left: w468 -> [w494]
              shift-right: [w486] -> w470
              shift-left: w472 -> [w482]
              shift-right: [w487] -> w471
              shift-left: w473 -> [w483]
              shift-right: [w481] -> _
              shift-left: w467 -> [w481]
              w496 = T11."Buffered" ("mode (standard)")
              n133 = TCP Read(connection ID=w483, bytes to read=w481, error in (no error)=w482, 7:w496) -> (connection ID out=w491:refnum<k5>, data out=w488:string, error out=w490:errorcluster)  [unwired: 1 in]
              n134 = Decimal String To Number(string=w488, default (0L)=u8 0 ("default (0 I32)")) -> (number=w485:u8)  [unwired: 1 in, 1 out]
              n135 = xnode "Read/Write Control"("FPGA VI Reference In"=w495, "error in"=w494, "analogue channel to write"=w485) -> ("FPGA VI Reference Out"=w493:refnum<k20>, "error out"=w492:errorcluster)
              n136 = TCP Read(connection ID=w491, bytes to read=w481, error in (no error)=w490, 7:w496) -> (connection ID out=w487:refnum<k5>, data out=w489:string, error out=w486:errorcluster)  [unwired: 1 in]
              n137 = Decimal String To Number(string=w489, default (0L)=u64 0 ("default (0 I32)")) -> (number=w484:u64)  [unwired: 1 in, 1 out]
              n138 = xnode "Read/Write Control"("FPGA VI Reference In"=w493, "error in"=w492, "analogue value to write"=w484) -> ("FPGA VI Reference Out"=w498:refnum<k20>, "error out"=w497:errorcluster)
            }
            n139 = xnode "Read/Write Control"("FPGA VI Reference In"=w463, "error in"=w462, "Trigger Write Analogue"=TRUE ("Digitals transfer done")) -> ("FPGA VI Reference Out"=w476:refnum<k20>, "error out"=w475:errorcluster)
          }
          frame 405 {
            # "Update Nr of repetitions"
            n140 = Unbundle By Name(w515) -> ("Message Length"=w499:u16)  [unwired: 2 out]
            n141 = TCP Read(connection ID=w514, bytes to read=w499, error in (no error)=w513, 7:T11."Buffered" ("mode (standard)")) -> (connection ID out=w508:refnum<k5>, data out=w502:string, error out=w500:errorcluster)  [unwired: 1 in]
            n142 = Decimal String To Number(string=w502, default (0L)=u32 0 ("default (0 I32)")) -> (number=w503:u32)  [unwired: 1 in, 1 out]
            n143 = xnode "Read/Write Control"("FPGA VI Reference In"=w512, "error in"=w505, "Nr of repetitions"=w503) -> ("FPGA VI Reference Out"=w506:refnum<k20>, "error out"=w501:errorcluster)
            n144 = xnode "Read/Write Control"("FPGA VI Reference In"=w506, "error in"=w501, "Trigger Repetitions update"=TRUE ("Digitals transfer done")) -> ("FPGA VI Reference Out"=w511:refnum<k20>, "error out"=w510:errorcluster)
          }
          frame 406 {
            w535 = u16 0 ("default (0 I32)")
            w550 = T11."Buffered" ("mode (standard)")
            # "Update Indexes"
            n145 = Unbundle By Name(w559) -> ("Number of Messages"=w529:u32, "Message Length"=w528:u16)
            n146 = TCP Read(connection ID=w533, bytes to read=w528, error in (no error)=w532, 7:w550) -> (connection ID out=w553:refnum<k5>, data out=w556:string, error out=w546:errorcluster)  [unwired: 1 in]
            n147 = Decimal String To Number(string=w556, default (0L)=u32 0 ("default (0 I32)")) -> (number=w552:u32)  [unwired: 1 in, 1 out]
            n148 = xnode "Read/Write Control"("FPGA VI Reference In"=w525, "error in"=w524, "indexesAddress"=w552) -> ("FPGA VI Reference Out"=w542:refnum<k20>, "error out"=w541:errorcluster)
            n149 = TCP Read(connection ID=w553, bytes to read=w528, error in (no error)=w546, 7:w550) -> (connection ID out=w551:refnum<k5>, data out=w555:string, error out=w545:errorcluster)  [unwired: 1 in]
            n150 = Decimal String To Number(string=w555, default (0L)=w535) -> (number=w549:u16)  [unwired: 1 in, 1 out]
            n151 = TCP Read(connection ID=w551, bytes to read=w528, error in (no error)=w545, 7:w550) -> (connection ID out=w543:refnum<k5>, data out=w554:string, error out=w544:errorcluster)  [unwired: 1 in]
            n152 = Decimal String To Number(string=w554, default (0L)=w535) -> (number=w547:u16)  [unwired: 1 in, 1 out]
            n153 = Bundle(w549, w547) -> (w548:cluster{u16, u16})  [unwired: 1 in]
            "output cluster 406" <- w548
            n154 = Subtract(x=w529, y=3) -> (x-y=w518:u32)
            n155 = xnode "Read/Write Control"("FPGA VI Reference In"=w542, "error in"=w541, "digital Indexes"=w548) -> ("FPGA VI Reference Out"=w540:refnum<k20>, "error out"=w539:errorcluster)
            n156 = Divide(x=w518, y=u32 2) -> (x/y=w519:fxp<+,8,8>)
            n157 = Initialize Array(u16 0, 0 ("dimension size")) -> (w522:u16[])
            n158 = for {
              N: w519 -> [_]
              shift-right: [w574] -> w531
              shift-left: w543 -> [w575]
              shift-right: [w576] -> w530
              shift-left: w544 -> [w578]
              shift-right: [w570] -> _
              shift-left: w528 -> [w570]
              shift-right: [w566] -> w521
              shift-left: w522 -> [w569]
              i -> [w563]
              w571 = u16 0 ("default (0 I32)")
              w579 = T11."Standard" ("mode (standard)")
              n159 = TCP Read(connection ID=w575, bytes to read=w570, error in (no error)=w578, 7:w579) -> (connection ID out=w580:refnum<k5>, data out=w573:string, error out=w577:errorcluster)  [unwired: 1 in]
              n160 = Multiply(x=2, y=w563) -> (x*y=w562:i32)
              n161 = Decimal String To Number(string=w573, default (0L)=w571) -> (number=w568:u16)  [unwired: 1 in, 1 out]
              n162 = Insert Into Array(array=w569, index=w562, new element=w568) -> (w567:u16[])
              n163 = Increment(x=w562) -> (x+1=w564:i32)
              n164 = TCP Read(connection ID=w580, bytes to read=w570, error in (no error)=w577, 7:w579) -> (connection ID out=w574:refnum<k5>, data out=w572:string, error out=w576:errorcluster)  [unwired: 1 in]
              n165 = Decimal String To Number(string=w572, default (0L)=w571) -> (number=w561:u16)  [unwired: 1 in, 1 out]
              n166 = Insert Into Array(array=w567, index=w564, new element=w561) -> (w566:u16[])
            }
            n167 = Array To Cluster(array=w521) -> (cluster=w538:T1)
            "cluster 406" <- w538
            n168 = xnode "Read/Write Control"("FPGA VI Reference In"=w540, "error in"=w539, "analogue Indexes"=w538) -> ("FPGA VI Reference Out"=w558:refnum<k20>, "error out"=w557:errorcluster)
            n169 = xnode "Read/Write Control"("FPGA VI Reference In"=w558, "error in"=w557, "Trigger Indexes Write"=TRUE) -> ("FPGA VI Reference Out"=w527:refnum<k20>, "error out"=w526:errorcluster)
          }
          frame 407 {
            # "initProfile"
            n170 = Unbundle By Name(w604) -> ("Message Length"=w581:u16)  [unwired: 2 out]
            n171 = TCP Read(connection ID=w603, bytes to read=w581, error in (no error)=w602, 7:T11."Buffered" ("mode (standard)")) -> (connection ID out=w597:refnum<k5>, data out=w591:string, error out=w586:errorcluster)  [unwired: 1 in]
            n172 = Decimal String To Number(string=w591, default (0L)=u32 0 ("default (0 I32)")) -> (number=w592:u32)  [unwired: 1 in, 1 out]
            n173 = xnode "Read/Write Control"("FPGA VI Reference In"=w601, "error in"=w594, "Nr of repetitions"=w592) -> ("FPGA VI Reference Out"=w595:refnum<k20>, "error out"=w589:errorcluster)
            n174 = TCP Read(connection ID=w597, bytes to read=w581, error in (no error)=w586) -> (connection ID out=w587:refnum<k5>, data out=w582:string, error out=w585:errorcluster)  [unwired: 2 in]
            n175 = Decimal String To Number(string=w582, default (0L)=u32 0 ("default (0 I32)")) -> (number=w583:u32)  [unwired: 1 in, 1 out]
            n176 = xnode "Read/Write Control"("FPGA VI Reference In"=w595, "error in"=w589, "Repetition timing"=w583) -> ("FPGA VI Reference Out"=w590:refnum<k20>, "error out"=w588:errorcluster)
            n177 = xnode "Read/Write Control"("FPGA VI Reference In"=w590, "error in"=w588, "Trigger Repetitions update"=TRUE ("Digitals transfer done")) -> ("FPGA VI Reference Out"=w600:refnum<k20>, "error out"=w599:errorcluster)
          }
          frame 408 {
            # "Trigger Experiment"
            n178 = Unbundle By Name(w613) -> ()  [unwired: 3 out]
            n179 = xnode "Read/Write Control"("FPGA VI Reference In"=w610, "error in"=w606, "Trigger Execute Experiment"=TRUE ("Digitals transfer done")) -> ("FPGA VI Reference Out"=w609:refnum<k20>, "error out"=w608:errorcluster)
          }
          frame 413 {
            n180 = Unbundle By Name(w629) -> ("Number of Messages"=w620:u32, "Message Length"=w619:u16)  [unwired: 1 out]
            n181 = for {
              N: w620 -> [_]
              shift-right: [w638] -> w624
              shift-left: w622 -> [w641]
              shift-right: [w637] -> w623
              shift-left: w621 -> [w640]
              shift-right: [w635] -> w615
              shift-left: i32[] [] -> [w636]
              shift-right: [w632] -> _
              shift-left: w619 -> [w632]
              n182 = TCP Read(connection ID=w641, bytes to read=w632, error in (no error)=w640, 7:T11."Buffered" ("mode (standard)")) -> (connection ID out=w638:refnum<k5>, data out=w633:string, error out=w637:errorcluster)  [unwired: 1 in]
              n183 = Decimal String To Number(string=w633, default (0L)=u64 0 ("default (0 I32)")) -> (number=w634:u64)  [unwired: 1 in, 1 out]
              n184 = Build Array (concatenate)(w636, w634) -> (w635:u64[])
            }
            n185 = xnode "Read/Write Control"("FPGA VI Reference In"=w616, "Take Snap  array"=w615) -> ("FPGA VI Reference Out"=w617:refnum<k20>)  [unwired: 1 in, 1 out]
            n186 = xnode "Read/Write Control"("FPGA VI Reference In"=w617, "error in"=w625, "Trigger Take Snap"=TRUE ("Digitals transfer done")) -> ("FPGA VI Reference Out"=w628:refnum<k20>, "error out"=w627:errorcluster)
          }
          frame 409 {
            # "Flush FIFOs"
            n187 = Unbundle By Name(w649) -> ()  [unwired: 3 out]
            n188 = xnode "Read/Write Control"("FPGA VI Reference In"=w646, "error in"=w642, "Trigger flush FIFOs"=TRUE ("Digitals transfer done")) -> ("FPGA VI Reference Out"=w645:refnum<k20>, "error out"=w644:errorcluster)
          }
        }
        n189 = xnode "Invoke Method"("FPGA VI Reference In"=w344, "error in"=w327, "IRQ Number(s)"=w324, "Timeout (ms)"=10000) -> ("FPGA VI Reference Out"=w329:refnum<k20>, "error out"=w326:errorcluster)  [unwired: 2 out]
        n190 = xnode "Read/Write Control"("FPGA VI Reference In"=w329, "error in"=w326) -> ("FPGA VI Reference Out"=w337:refnum<k20>, "error out"=w331:errorcluster, "Error code"=w335:u8)
        n191 = Not Equal To 0?(x=w335) -> (x != 0?=w336:bool)
        n192 = case shown="True" w336 {
          tunnel: [w348 w351] -> w322
          tunnel: w331 -> [w348 w352]
          tunnel: w335 -> [_ w349]
          frame False {
          }
          frame True {
            n193 = call <vilib>:"Error Cluster From Error Code.vi"("error in (no error)"=w352, "error message (\"\")"="FPGA error" ("error message (\"\")"), "error code (0)"=w349) -> ("error out"=w351:errorcluster)  [unwired: 6 in]
          }
        }
        n194 = xnode "Invoke Method"("FPGA VI Reference In"=w337, "error in"=w322, "IRQ Number(s)"=w324) -> ("FPGA VI Reference Out"=w325:refnum<k20>, "error out"=w323:errorcluster)
      }
      frame "Sending Async Command" {
        n195 = case shown="0, Default" w671 {
          tunnel: [w683 w691 w700 w707 w722] -> w670
          tunnel: w669 -> [w683 w691 w700 w707 w722]
          tunnel: [w682 w690 w699 w706 w721] -> w658
          tunnel: w668 -> [w682 w690 w699 w706 w721]
          tunnel: [w677 w688 w697 w705 w719] -> w667
          tunnel: w651 -> [w677 w689 w698 w705 w720]
          tunnel: [w681 w687 w696 w704 w718] -> w659
          tunnel: w666 -> [w681 w685 w695 w704 w717]
          tunnel: w665 -> [w679 w692 w701 w708 w723]
          tunnel: [w680 w693 w702 w709 w724] -> w660
          tunnel: w664 -> [w680 w693 w702 w709 w724]
          tunnel: [T5."Idle" ("RT-host Main State") T5."Idle" ("RT-host Main State") T5."Reset" ("RT-host Main State") T5."Reset" ("RT-host Main State") T5."Idle" ("RT-host Main State")] -> w662
          frame 0, Default {
            n196 = Unbundle By Name(w679) -> ()  [unwired: 3 out]
          }
          frame 301 {
            # "Abort FPGA"
            n197 = Unbundle By Name(w692) -> ()  [unwired: 3 out]
            n198 = xnode "Read/Write Control"("FPGA VI Reference In"=w689, "error in"=w685, "Trigger Abort"=TRUE ("Digitals transfer done")) -> ("FPGA VI Reference Out"=w688:refnum<k20>, "error out"=w687:errorcluster)
          }
          frame 302 {
            # "Restart FPGA and RT-Host"
            n199 = Unbundle By Name(w701) -> ()  [unwired: 3 out]
            n200 = xnode "Invoke Method"("FPGA VI Reference In"=w698, "error in"=w695) -> ("FPGA VI Reference Out"=w697:refnum<k20>, "error out"=w696:errorcluster)
          }
          frame 303 {
            # "Restart RT-Host"
            n201 = Unbundle By Name(w708) -> ()  [unwired: 3 out]
          }
          frame 304 {
            # "Restart FPGA"
            n202 = Unbundle By Name(w723) -> ()  [unwired: 3 out]
            n203 = flat-sequence {
              tunnel: w717 -> [w726]
              tunnel: w720 -> [w727]
              tunnel: [w727] -> w711
              tunnel: [w726] -> w710
              tunnel: [w730] -> w713
              tunnel: [w729] -> w712
              tunnel: w711 -> [w730]
              tunnel: w710 -> [w729]
              tunnel: [w733] -> w715
              tunnel: [w732] -> w714
              tunnel: w713 -> [w734]
              tunnel: w712 -> [w731]
              tunnel: [w736] -> w718
              tunnel: [w737] -> w719
              tunnel: w715 -> [w737]
              tunnel: w714 -> [w736]
              frame #0 {
                n204 = local write "Run Status reporter"(FALSE) -> ()
              }
              frame #1 {
                n205 = local read "UDP refresh rate"() -> (w728:u16)
                n206 = Wait (ms)(milliseconds to wait=w728) -> ()  [unwired: 1 out]
              }
              frame #2 {
                n207 = xnode "Invoke Method"("FPGA VI Reference In"=w734, "error in"=w731) -> ("FPGA VI Reference Out"=w733:refnum<k20>, "error out"=w732:errorcluster)
              }
              frame #3 {
                n208 = local write "Run Status reporter"(TRUE) -> ()
              }
            }
          }
        }
        n209 = xnode "Read/Write Control"("FPGA VI Reference In"=w667, "error in"=w659) -> ("FPGA VI Reference Out"=w655:refnum<k20>, "error out"=w656:errorcluster, "Error code"=w653:u8)
        n210 = Not Equal To 0?(x=w653) -> (x != 0?=w657:bool)
        n211 = case shown="True" w657 {
          tunnel: [w672 w675] -> w654
          tunnel: w656 -> [w672 w676]
          tunnel: w653 -> [_ w673]
          frame False {
          }
          frame True {
            n212 = call <vilib>:"Error Cluster From Error Code.vi"("error in (no error)"=w676, "error message (\"\")"="FPGA error" ("error message (\"\")"), "error code (0)"=w673) -> ("error out"=w675:errorcluster)  [unwired: 6 in]
          }
        }
      }
    }
    n213 = Merge Errors(w108, w109, w112) -> (w102:errorcluster)
    n214 = Unbundle By Name(w102) -> ("status"=w104:bool)
    n215 = case shown="False" w103 {
      tunnel: w106 -> [w126 w134]
      tunnel: [w126 w133] -> w105
      tunnel: [w125 w132] -> w107
      tunnel: w102 -> [_ w131]
      tunnel: w108 -> [w125 w130]
      frame False {
      }
      frame True {
        n216 = Flatten To JSON(anything=w131) -> (JSON string=w129:string)  [unwired: 2 in, 1 out]
        n217 = String Length(string=w129) -> (length=w128:i32)
        n218 = Number To Decimal String(number=w128, width (-)=i16 4) -> ()  [unwired: 1 out]
        n219 = TCP Write(connection ID=w134, data in=w129, error in (no error)=w130) -> (connection ID out=w133:refnum<k5>, error out=w132:errorcluster)  [unwired: 1 in, 1 out]
      }
    }
    n220 = case shown="True" w104 {
      tunnel: [w136 w141] -> w113
      tunnel: w102 -> [w136 w140]
      tunnel: w101 -> [w135 w138]
      tunnel: [w135 w137] -> w100
      frame False {
      }
      frame True {
        n221 = Unbundle By Name(w140) -> ("code"=w139:i32)
        n222 = case shown="66" w139 {
          tunnel: w138 -> [w142 _]
          tunnel: [w142 T5."Start" ("RT-host Main State")] -> w137
          frame 0, Default {
          }
          frame 66 {
          }
        }
        n223 = call <vilib>:"Clear Errors.vi"("error in (no error)"=w140) -> ("error out"=w141:errorcluster)  [unwired: 5 in, 1 out]
        "error out" <- w140
      }
    }
    n224 = call <vilib>:"Clear Errors.vi"("error in (no error)"=w107) -> ("error out"=w110:errorcluster)  [unwired: 5 in, 1 out]
    n225 = call <vilib>:"Clear Errors.vi"("error in (no error)"=w109) -> ("error out"=w111:errorcluster)  [unwired: 5 in, 1 out]
    "RT-host Action State" <- w115
  }
